vi "Get Target Location.vi"(11 "RTTarget in":refnum<class "RTTarget.lvclass">) -> (3 "target location":string)   [LabVIEW 2020, in "NI_TargetHelper.lvlib" / "RTTarget.lvclass"]
uses:
  <vilib>/TargetSupport/NI_TargetHelper/RTTarget/RTTarget.lvclass
  <vilib>/TargetSupport/NI_TargetHelper/RTTarget/RTTarget.lvclass/RTTarget.ctl
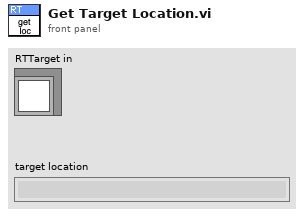
[diagram p1: front panel]
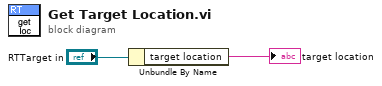
[diagram p0: block diagram]
diagram:
  n1 = Unbundle By Name("RTTarget in") -> ("target location"=→"target location":string)
